vi "set enable autogain.vi"(8 "error in (no error)":errorcluster, 11 "Thorcam in":refnum<class "Thorcam.lvclass">) -> (0 "error out":errorcluster, 3 "Thorcam out":refnum<class "Thorcam.lvclass">)   [LabVIEW 2012, in "Thorcam.lvclass"]
uses:
  Thorcam.lvclass
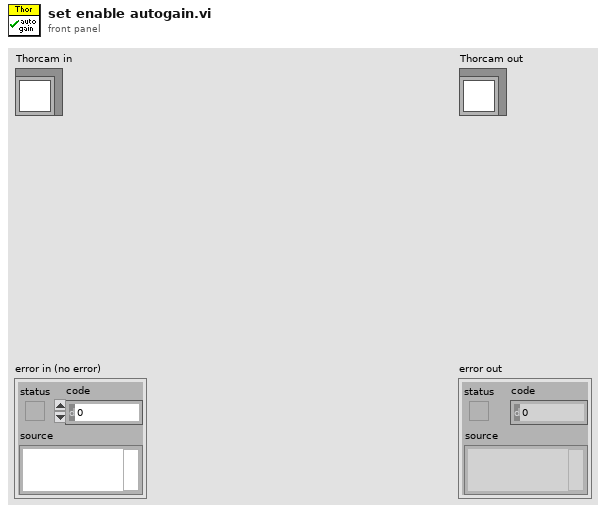
[diagram p1: front panel]
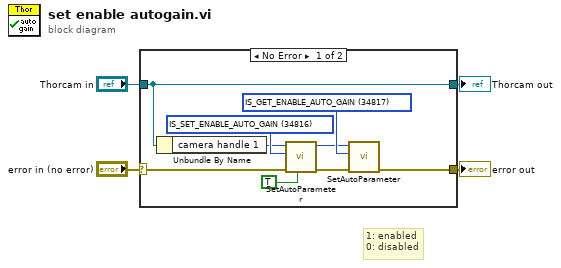
[diagram p0: block diagram]
diagram:
  # "1: enabled\n0: disabled"
  n1 = case shown="No Error" "error in (no error)" {
    selector: "error in (no error)" -> [w7 w15]
    tunnel: [w6 w15] -> w3
    tunnel: [w5 w14] -> w1
    tunnel: "Thorcam in" -> [w5 w14]
    frame No Error {
      w12 = 34817 items=["IS_SET_ENABLE_AUTO_GAIN"=34816, "IS_GET_ENABLE_AUTO_GAIN"=34817, "IS_SET_ENABLE_AUTO_SHUTTER"=34818, "IS_GET_ENABLE_AUTO_SHUTTER"=34819, "IS_SET_ENABLE_AUTO_WHITEBALANCE"=34820, "IS_GET_ENABLE_AUTO_WHITEBALANCE"=34821, "IS_SET_ENABLE_AUTO_FRAMERATE"=34822, "IS_GET_ENABLE_AUTO_FRAMERATE"=34823, "IS_SET_AUTO_REFERENCE"=32768, "IS_GET_AUTO_REFERENCE"=32769, "IS_SET_AUTO_GAIN_MAX"=32770, "IS_GET_AUTO_GAIN_MAX"=32771, "IS_SET_AUTO_SHUTTER_MAX"=32772, "IS_GET_AUTO_SHUTTER_MAX"=32773, "IS_SET_AUTO_SPEED"=32774, "IS_GET_AUTO_SPEED"=32775, "IS_SET_AUTO_WB_OFFSET"=32776, "IS_GET_AUTO_WB_OFFSET"=32777, "IS_SET_AUTO_WB_GAIN_RANGE"=32778, "IS_GET_AUTO_WB_GAIN_RANGE"=32779, "IS_SET_AUTO_WB_SPEED"=32780, "IS_GET_SUTO_WB_SPEED"=32781, "IS_SET_AUTO_WB_ONCE"=32782, "IS_GET_AUTO_WB_ONCE"=32783] ("Param")
      w9 = 34816 items=["IS_SET_ENABLE_AUTO_GAIN"=34816, "IS_GET_ENABLE_AUTO_GAIN"=34817, "IS_SET_ENABLE_AUTO_SHUTTER"=34818, "IS_GET_ENABLE_AUTO_SHUTTER"=34819, "IS_SET_ENABLE_AUTO_WHITEBALANCE"=34820, "IS_GET_ENABLE_AUTO_WHITEBALANCE"=34821, "IS_SET_ENABLE_AUTO_FRAMERATE"=34822, "IS_GET_ENABLE_AUTO_FRAMERATE"=34823, "IS_SET_AUTO_REFERENCE"=32768, "IS_GET_AUTO_REFERENCE"=32769, "IS_SET_AUTO_GAIN_MAX"=32770, "IS_GET_AUTO_GAIN_MAX"=32771, "IS_SET_AUTO_SHUTTER_MAX"=32772, "IS_GET_AUTO_SHUTTER_MAX"=32773, "IS_SET_AUTO_SPEED"=32774, "IS_GET_AUTO_SPEED"=32775, "IS_SET_AUTO_WB_OFFSET"=32776, "IS_GET_AUTO_WB_OFFSET"=32777, "IS_SET_AUTO_WB_GAIN_RANGE"=32778, "IS_GET_AUTO_WB_GAIN_RANGE"=32779, "IS_SET_AUTO_WB_SPEED"=32780, "IS_GET_SUTO_WB_SPEED"=32781, "IS_SET_AUTO_WB_ONCE"=32782, "IS_GET_AUTO_WB_ONCE"=32783] ("Param")
      n2 = Unbundle By Name(w5) -> ("camera handle 1"=w8:u32)
      n3 = call <instrlib>:"SetAutoParameter.vi"("enable"=TRUE, "error in"=w7, "Param"=w9, "Camera Handle In"=w8) -> ("error out"=w10:errorcluster, "Camera Handle Out"=w11:u32)  [unwired: 5 in, 1 out]
      n4 = call <instrlib>:"SetAutoParameter.vi"("error in"=w10, "Param"=w12, "Camera Handle In"=w11) -> ("error out"=w6:errorcluster)  [unwired: 6 in, 2 out]
    }
    frame Error {
    }
  }
  "error out" <- w3
  "Thorcam out" <- w1
